vi "Problem2.5-TestProgram.vi"() -> ()   [LabVIEW 2019]
panel:
  in  "Loop Delay (ms)":dbl=100.0
  out "Elapsed Time (s)":dbl
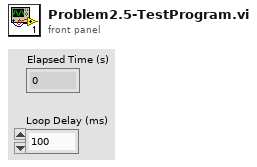
[diagram p1: front panel]
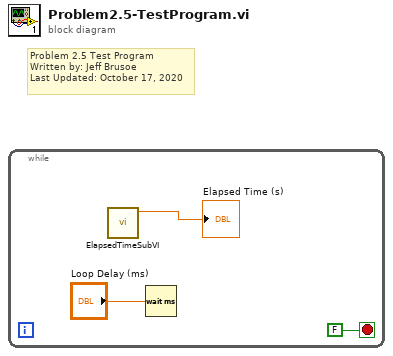
[diagram p0: block diagram]
diagram:
  # "Problem 2.5 Test Program\nWritten by: Jeff Brusoe\nLast Updated: October 17, 2020"
  n1 = while {
    stop <- FALSE stop-if-true
    n2 = call "ElapsedTimeSubVI.vi"() -> ("Elapsed Time (s)"=→"Elapsed Time (s)":dbl)  [unwired: 11 in]
    n3 = Wait (ms)(milliseconds to wait="Loop Delay (ms)") -> ()  [unwired: 1 out]
  }
